vi "DB to Tree.vi"() -> ()   [LabVIEW 2020]
uses:
  <vilib>/addons/database/NI_Database_API.lvlib
  <vilib>/addons/database/Connection.llb/Conn Execute.vi
  <vilib>/addons/database/Recordset.llb/Rec Fetch Recordset Data (R).vi
  <vilib>/addons/database/Recordset.llb/Rec Destroy - Connection.vi
  <vilib>/addons/database/_DB Variant To Data/Database Variant To Data.xnode
  <vilib>/addons/database/Connection.llb/DB Tools Open Connec (String).vi
panel:
  out "All Tags 2":string[](array[string])
  in  "stop":bool
  out "Column":string[](array[string])
  out "Table":string[](array[string])
  out "DB":string[](array[string])
  out "All Tags":string[](array[string])
  in  "Tree":string[](tree)
  out "data":string[][](array[string])
  out "error out 2":errorcluster
  out "error out":errorcluster
  out "String":string
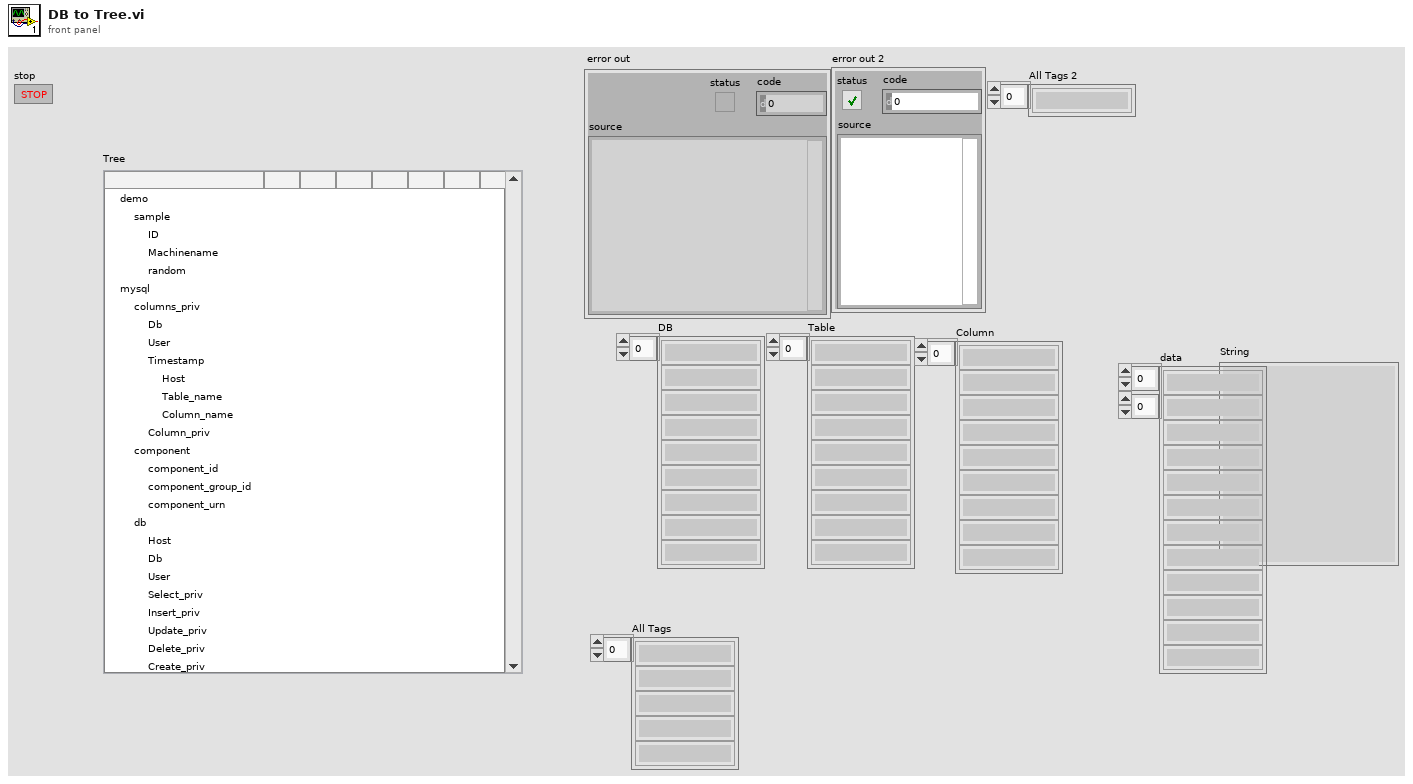
[diagram p1: front panel]
types:
  T1 = cluster{"Left Cell String":string, "Child Text":string[], "Child Tag":string, "Item Indent":i32, "Child Only?":bool, "Glyph Index":i32}[]
  T2 = cluster{"Left Cell String":string, "Child Text":string[], "Child Tag":string, "Item Indent":i32, "Child Only?":bool, "Glyph Index":i32}
  T3 = typedef "NI_Database_API.lvlib/Conn ObjectReference.ctl" = refnum<k1>
  T4 = typedef "NI_Database_API.lvlib/Rec ObjectReference.ctl" = refnum<k1>
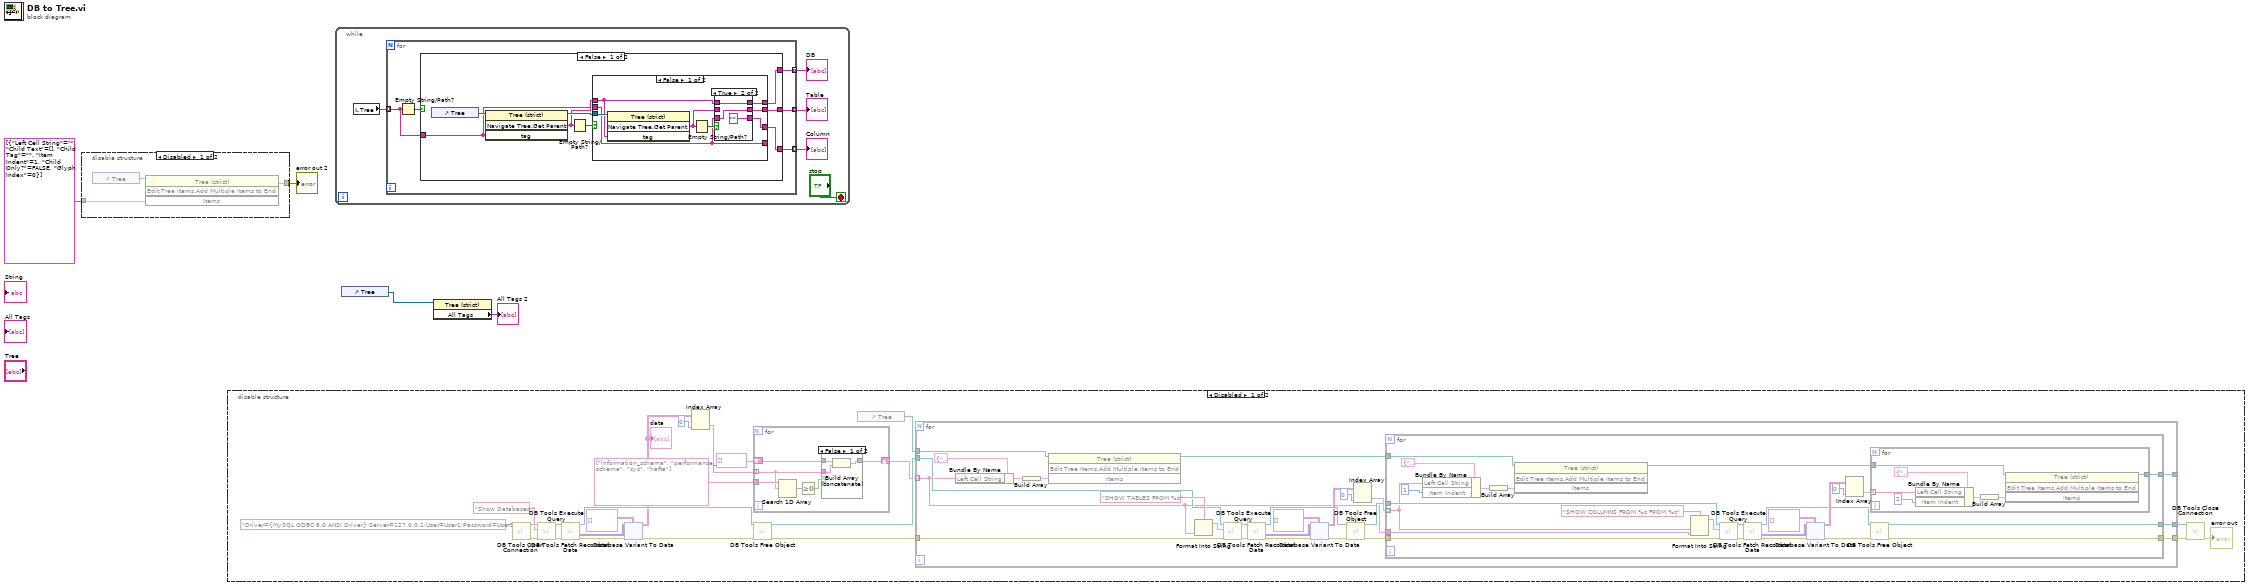
[diagram p0: block diagram]
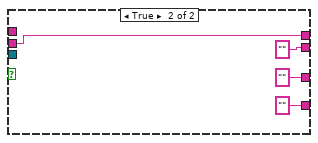
[diagram p3: hidden frame]
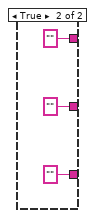
[diagram p4: hidden frame]
diagram:
  n1 = disable-structure shown="Disabled" {
    disable-tunnel: T1 [{"Left Cell String"="", "Child Text"=[], "Child Tag"="", "Item Indent"=1, "Child Only?"=FALSE, "Glyph Index"=0}] ("Items") -> [w7 _]
    disable-tunnel: [w6 _] -> w3
    frame Disabled {
      n2 = control-ref of="Tree"() -> (w5:refnum<vi>)
      n3 = invoke on="Invoke Node" class="Tree (strict)" method="Edit Tree Items.Add Multiple Items to End"(reference=w5, "Items"=w7) -> (error out=w6:errorcluster)  [unwired: 2 in, 3 out]
    }
    frame Enabled {
    }
  }
  "error out 2" <- w3
  n4 = disable-structure shown="Disabled" {
    frame Disabled {
      n5 = call-poly <vilib>:"DB Tools Open Connection.vi"("connection information"="Driver={MySQL ODBC 8.0 ANSI Driver};Server=127.0.0.1;User=User1;Password=User1.;") -> ("error out"=w27:errorcluster, "connection reference"=w28:T3)  [unwired: 7 in]
      n6 = call-poly <vilib>:"DB Tools Execute Query.vi"("error in (no error)"=w27, "SQL query"="Show Databases;", "connection reference"=w28) -> ("error out"=w24:errorcluster, "recordset reference"=w25:T4)  [unwired: 5 in]
      n7 = call-poly <vilib>:"DB Tools Fetch Recordset Data.vi"("error in (no error)"=w24, "recordset reference"=w25) -> ("error out"=w20:errorcluster, "recordset data"=w22:variant[][], "recordset reference out"=w23:T4)  [unwired: 3 in]
      n8 = xnode "Database Variant To Data"("database variant"=w22, "error in (no error)"=w20, "type"=string[][] []) -> ("data"=w18:string[][], "error out"=w19:errorcluster)
      "data" <- w18
      n9 = Index Array(array=w18, index (col)=0 ("disabled index (col)")) -> (element=w9:string[])  [unwired: 1 in]
      n10 = for {
        tunnel: w9 -> [w31] mode=indexing
        shift-right: [w33] -> w8
        shift-left: string[] [] -> [w32]
        tunnel: string[] ["information_schema", "performance_schema", "sys", "hafta"] -> [w36]
        n11 = Search 1D Array(1D array=w36, element=w31) -> (index of element=w35:i32)  [unwired: 1 in]
        n12 = Greater Or Equal To 0?(x=w35) -> (x >= 0?=w34:bool)
        n13 = case shown="False" w34 {
          tunnel: [w37 w40] -> w33
          tunnel: w32 -> [w38 w40]
          tunnel: w31 -> [w39 _]
          frame False {
            n14 = Build Array (concatenate)(w38, w39) -> (w37:string[])
          }
          frame True {
          }
        }
      }
      n15 = call-poly <vilib>:"DB Tools Free Object.vi"("error in (no error)"=w19, "recordset reference"=w23) -> ("error out"=w15:errorcluster, "connection reference"=w16:T3)  [unwired: 8 in]
      n16 = control-ref of="Tree"() -> (w10:refnum<vi>)
      n17 = for {
        tunnel: w16 -> [w63]
        tunnel: w15 -> [w62]
        tunnel: w10 -> [w65]
        tunnel: w8 -> [w42] mode=indexing
        tunnel: [w48] -> w14
        tunnel: [w47] -> w13
        tunnel: [w41] -> _
        n18 = Bundle By Name(cluster=T2 {"Left Cell String"="", "Child Text"=[], "Child Tag"="", "Item Indent"=0, "Child Only?"=FALSE, "Glyph Index"=0} ("Item"), "Left Cell String"=w42) -> (w45:T2)
        n19 = Build Array(w45) -> (w44:T1)
        n20 = invoke on="Invoke Node" class="Tree (strict)" method="Edit Tree Items.Add Multiple Items to End"(reference=w65, "Items"=w44) -> (reference out=w43:refnum<vi>)  [unwired: 2 in, 3 out]
        n21 = Format Into String(format string="SHOW TABLES FROM %s", w42) -> (resulting string=w61:string)  [unwired: 2 in, 1 out]
        n22 = call-poly <vilib>:"DB Tools Execute Query.vi"("error in (no error)"=w62, "SQL query"=w61, "connection reference"=w63) -> ("error out"=w59:errorcluster, "recordset reference"=w60:T4)  [unwired: 5 in]
        n23 = call-poly <vilib>:"DB Tools Fetch Recordset Data.vi"("error in (no error)"=w59, "recordset reference"=w60) -> ("error out"=w55:errorcluster, "recordset data"=w56:variant[][], "recordset reference out"=w58:T4)  [unwired: 3 in]
        n24 = xnode "Database Variant To Data"("database variant"=w56, "error in (no error)"=w55, "type"=string[][] []) -> ("data"=w53:string[][], "error out"=w54:errorcluster)
        n25 = call-poly <vilib>:"DB Tools Free Object.vi"("error in (no error)"=w54, "recordset reference"=w58) -> ("error out"=w49:errorcluster, "connection reference"=w50:T3)  [unwired: 8 in]
        n26 = Index Array(array=w53, index (col)=0 ("disabled index (col)")) -> (element=w51:string[])  [unwired: 1 in]
        n27 = for {
          tunnel: w51 -> [w116] mode=indexing
          tunnel: w50 -> [w123]
          tunnel: w49 -> [w122]
          tunnel: [w121] -> w48
          tunnel: [w120] -> w47
          tunnel: w43 -> [w113]
          tunnel: w42 -> [w111]
          tunnel: [w110] -> w41
          n28 = Bundle By Name(cluster=T2 {"Left Cell String"="", "Child Text"=[], "Child Tag"="", "Item Indent"=0, "Child Only?"=FALSE, "Glyph Index"=0} ("Item"), "Left Cell String"=w116, "Item Indent"=1) -> (w119:T2)
          n29 = Build Array(w119) -> (w117:T1)
          n30 = invoke on="Invoke Node" class="Tree (strict)" method="Edit Tree Items.Add Multiple Items to End"(reference=w113, "Items"=w117) -> (reference out=w112:refnum<vi>)  [unwired: 2 in, 3 out]
          n31 = Format Into String(format string="SHOW COLUMNS FROM %s FROM %s", w116, w111) -> (resulting string=w125:string)  [unwired: 2 in, 1 out]
          n32 = call-poly <vilib>:"DB Tools Execute Query.vi"("error in (no error)"=w122, "SQL query"=w125, "connection reference"=w123) -> ("error out"=w127:errorcluster, "recordset reference"=w126:T4)  [unwired: 5 in]
          n33 = call-poly <vilib>:"DB Tools Fetch Recordset Data.vi"("error in (no error)"=w127, "recordset reference"=w126) -> ("error out"=w131:errorcluster, "recordset data"=w130:variant[][], "recordset reference out"=w128:T4)  [unwired: 3 in]
          n34 = xnode "Database Variant To Data"("database variant"=w130, "error in (no error)"=w131, "type"=string[][] []) -> ("data"=w133:string[][], "error out"=w132:errorcluster)
          n35 = Index Array(array=w133, index (col)=0 ("disabled index (col)")) -> (element=w114:string[])  [unwired: 1 in]
          n36 = for {
            tunnel: w114 -> [w137] mode=indexing
            tunnel: w112 -> [w136]
            tunnel: [w135] -> w110
            n37 = Bundle By Name(cluster=T2 {"Left Cell String"="", "Child Text"=[], "Child Tag"="", "Item Indent"=0, "Child Only?"=FALSE, "Glyph Index"=0} ("Item"), "Left Cell String"=w137, "Item Indent"=2) -> (w138:T2)
            n38 = Build Array(w138) -> (w140:T1)
            n39 = invoke on="Invoke Node" class="Tree (strict)" method="Edit Tree Items.Add Multiple Items to End"(reference=w136, "Items"=w140) -> (reference out=w135:refnum<vi>)  [unwired: 2 in, 3 out]
          }
          n40 = call-poly <vilib>:"DB Tools Free Object.vi"("error in (no error)"=w132, "recordset reference"=w128) -> ("error out"=w121:errorcluster, "connection reference"=w120:T3)  [unwired: 8 in]
        }
      }
      n41 = call <vilib>:"DB Tools Close Connection.vi"("error in (no error)"=w14, "connection reference"=w13) -> ("error out"=→"error out":errorcluster)  [unwired: 5 in]
    }
    frame Enabled {
    }
  }
  n42 = while {
    stop <- "stop" stop-if-true
    n43 = local read "Tree"() -> (w234:string[])
    n44 = for {
      tunnel: w234 -> [w236] mode=indexing
      tunnel: [w238] -> w233 mode=indexing
      tunnel: [w237] -> w232 mode=indexing
      tunnel: [w235] -> w231 mode=indexing
      n45 = Empty String/Path?(string/path=w236) -> (empty?=w239:bool)
      n46 = case shown="False" w239 {
        tunnel: w236 -> [w241 _]
        tunnel: [w245 "" ("Navigate Tree:Get Parent")] -> w238
        tunnel: [w242 "" ("Navigate Tree:Get Parent")] -> w237
        tunnel: [w240 ""] -> w235
        frame False {
          n47 = control-ref of="Tree"() -> (w247:refnum<vi>)
          n48 = invoke class="Tree (strict)" method="Navigate Tree.Get Parent"(reference=w247, "tag"=w241) -> (reference out=w246:refnum<vi>, "Navigate Tree:Get Parent"=w244:string)  [unwired: 2 in, 2 out]
          n49 = Empty String/Path?(string/path=w244) -> (empty?=w243:bool)
          n50 = case shown="False" w243 {
            tunnel: w246 -> [w255 _]
            tunnel: [w252 w265] -> w245
            tunnel: w244 -> [w251 _]
            tunnel: [w250 "" ("Navigate Tree:Get Parent")] -> w242
            tunnel: w241 -> [w249 w265]
            tunnel: [w249 ""] -> _
            tunnel: [w248 ""] -> w240
            frame False {
              n51 = invoke class="Tree (strict)" method="Navigate Tree.Get Parent"(reference=w255, "tag"=w251) -> ("Navigate Tree:Get Parent"=w253:string)  [unwired: 2 in, 3 out]
              n52 = Empty String/Path?(string/path=w253) -> (empty?=w254:bool)
              n53 = case shown="True" w254 {
                tunnel: w253 -> [w258 _]
                tunnel: [w258 w261] -> w252
                tunnel: w251 -> [w257 w261]
                tunnel: [w257 w260] -> w250
                tunnel: w249 -> [w256 w260]
                tunnel: [w256 ""] -> w248
                frame False {
                }
                frame True {
                }
              }
            }
            frame True {
            }
          }
        }
        frame True {
        }
      }
    }
    "DB" <- w233
    "Table" <- w232
    "Column" <- w231
  }
  n54 = control-ref of="Tree"() -> (w1:refnum<vi>)
  n55 = property class="Tree (strict)"(reference=w1) -> ("All Tags"=→"All Tags 2":string[])  [unwired: 1 in, 2 out]
